vi "keccak.impl.vi"(11 "Array in":u64[](array[numeric])) -> (3 "Array out":u64[](array[numeric]))   [LabVIEW 2021]
uses:
  Step.4.5.6.7.Inputs.ctl
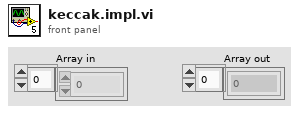
[diagram p1: front panel]
types:
  T1 = typedef "Step.4.5.6.7.Inputs.ctl" = cluster{"Left_Shift":i32, "State_Index":i32, "D_Index":i32}
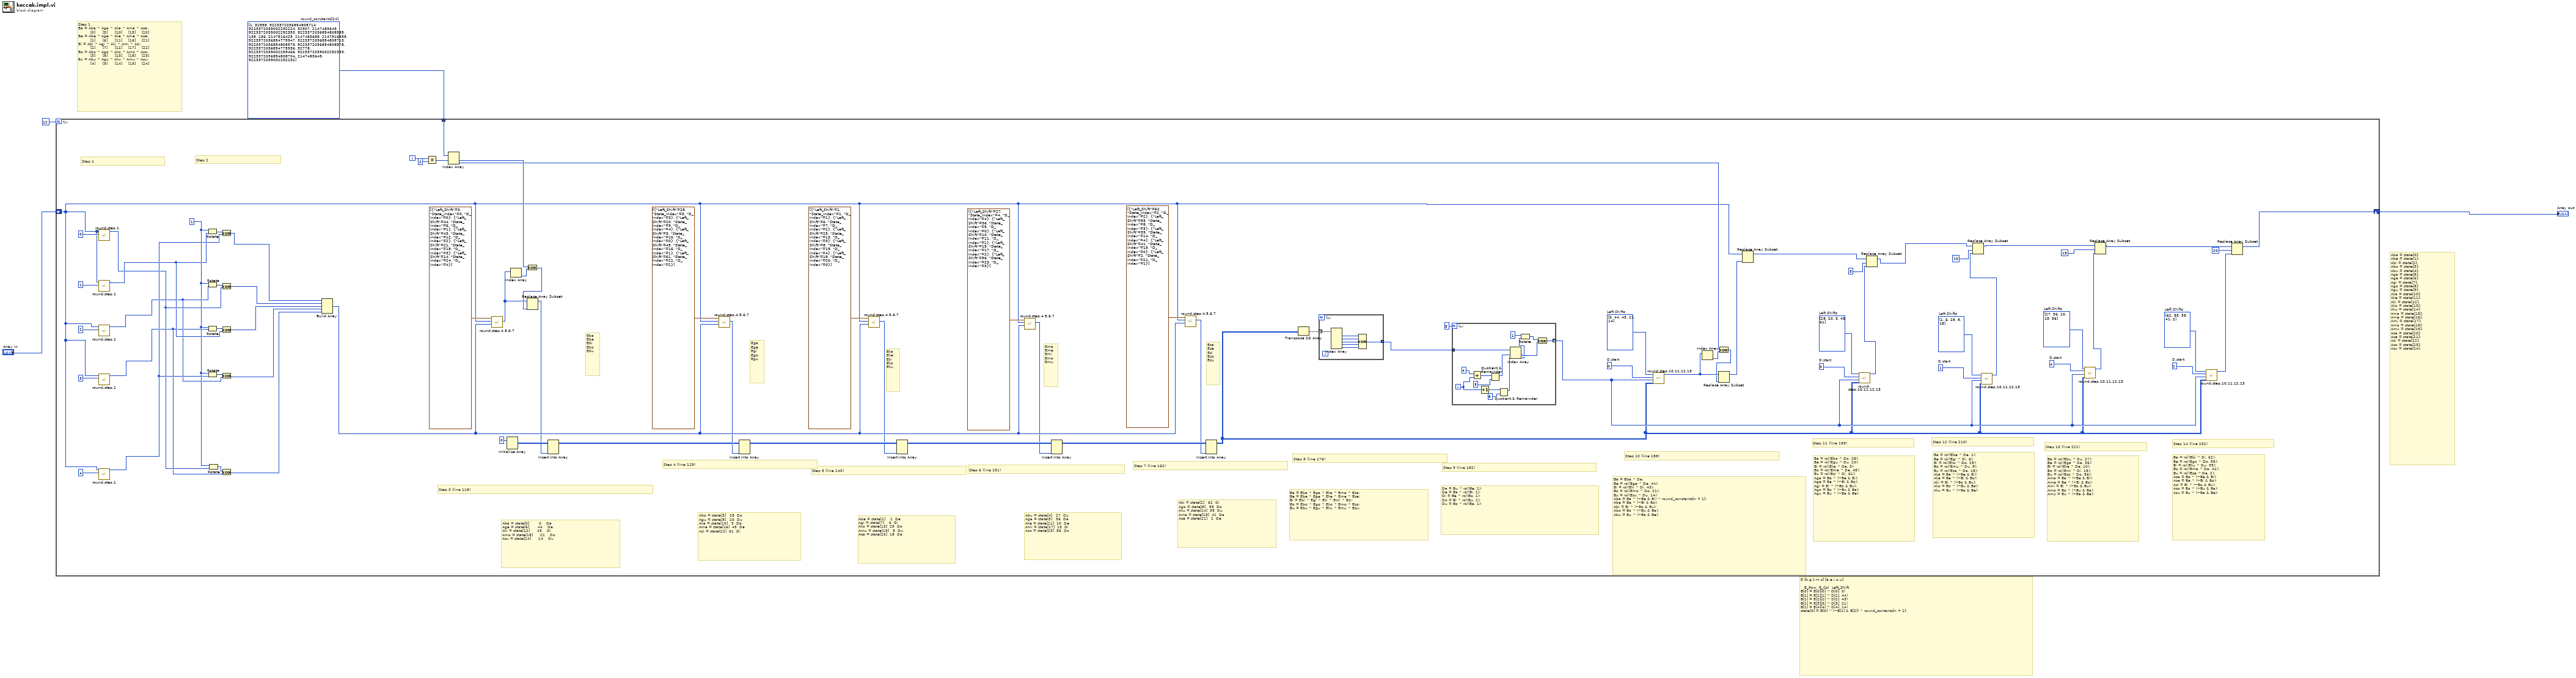
[diagram p0: block diagram]
diagram:
  w3 = u64[] [1, 32898, 9223372036854808714, 9223372039002292224, 32907, 2147483649, 9223372039002292353, 9223372036854808585, 138, 136, 2147516425, 2147483658, 2147516555, 9223372036854775947, 9223372036854808713, 9223372036854808579, 9223372036854808578, 9223372036854775936, 32778, 9223372039002259466, 9223372039002292353, 9223372036854808704, 2147483649, 9223372039002292232]  # round_constants[24]
  # "E [b,g,k,m,s] [a,e,i,o,u]\n\n   E_Row  E_Col  Left_Shift\nB[0] = E[0][0] ^ D[0], 0)\nB[1] = E[1][1] ^ D[1], 44)\nB[1] = E[2][2] ^ D[2], 43)\nB[1] = E[3][3] ^ D[3], 21)\nB[1] = E[4][4] ^ D[4], 14)\nstate[0] = B[0] ^ (~B[1] & B[2]) ^ round_contants[n + 1];"
  # "Aba = state[0];\nAbe = state[1];\nAbi = state[2];\nAbo = state[3];\nAbu = state[4];\nAga = state[5];\nAge = state[6];\nAgi = state[7];\nAgo = state[8];\nAgu = state[9];\nAka = state[10];\nAke = state[11];\nAki = state[12];\nAko = state[13];\nAku = state[14];\nAma = state[15];\nAme = state[16];\nAmi = state[17];\nAmo = state[18];\nAmu = state[19];\nAsa = state[20];\nAse = state[21];\nAsi = state[22];\nAso = state[23];\nAsu = state[24];"
  # "Step 1\nBa = Aba ^ Aga ^ Aka ^ Ama ^ Asa;\n          [0]      [5]      [10]     [15]     [20]\nBe = Abe ^ Age ^ Ake ^ Ame ^ Ase;\n          [1]      [6]      [11]     [16]     [21]\nBi = Abi ^ Agi ^ Aki ^ Ami ^ Asi;\n          [2]      [7]      [12]     [17]     [22]\nBo = Abo ^ Ago ^ Ako ^ Amo ^ Aso;\n          [3]      [8]      [13]     [18]     [23]\nBu = Abu ^ Agu ^ Aku ^ Amu ^ Asu;\n          [4]      [9]      [14]     [19]     [24]"
  n1 = for {
    N: 12 -> [_]
    tunnel: w3 -> [w65]
    shift-right: [w19] -> w4
    shift-left: "Array in" -> [w7]
    i -> [w84]
    w23 = 2  # D.start
    w22 = 4  # D.start
    w24 = i32[] [62, 55, 39, 41, 2]  # Left Shifts
    w25 = i32[] [27, 36, 10, 15, 56]  # Left Shifts
    w26 = 1  # D.start
    w27 = i32[] [1, 6, 25, 8, 18]  # Left Shifts
    w28 = 3  # D.start
    w29 = i32[] [28, 20, 3, 45, 61]  # Left Shifts
    w30 = 0  # D.start
    w35 = i32[] [0, 44, 43, 21, 14]  # Left Shifts
    w72 = i16 1 ("y")
    # "Ba = rol(Ebi ^ Di, 62);\nBe = rol(Ego ^ Do, 55);\nBi = rol(Eku ^ Du, 39);\nBo = rol(Ema ^ Da, 41);\nBu = rol(Ese ^ De, 2);\nAsa = Ba ^ (~Be & Bi);\nAse = Be ^ (~Bi & Bo);\nAsi = Bi ^ (~Bo & Bu);\nAso = Bo ^ (~Bu & Ba);\nAsu = Bu ^ (~Ba & Be);"
    # "Ba = rol(Ebu ^ Du, 27);\nBe = rol(Ega ^ Da, 36);\nBi = rol(Eke ^ De, 10);\nBo = rol(Emi ^ Di, 15);\nBu = rol(Eso ^ Do, 56);\nAma = Ba ^ (~Be & Bi);\nAme = Be ^ (~Bi & Bo);\nAmi = Bi ^ (~Bo & Bu);\nAmo = Bo ^ (~Bu & Ba);\nAmu = Bu ^ (~Ba & Be);"
    # "Step 14 (line 232)"
    # "Step 13 (line 221)"
    # "Ba = rol(Ebe ^ De, 1);\nBe = rol(Egi ^ Di, 6);\nBi = rol(Eko ^ Do, 25);\nBo = rol(Emu ^ Du, 8);\nBu = rol(Esa ^ Da, 18);\nAka = Ba ^ (~Be & Bi);\nAke = Be ^ (~Bi & Bo);\nAki = Bi ^ (~Bo & Bu);\nAko = Bo ^ (~Bu & Ba);\nAku = Bu ^ (~Ba & Be);"
    # "Step 12 (line 210)"
    # "Ba = rol(Ebo ^ Do, 28);\nBe = rol(Egu ^ Du, 20);\nBi = rol(Eka ^ Da, 3);\nBo = rol(Eme ^ De, 45);\nBu = rol(Esi ^ Di, 61);\nAga = Ba ^ (~Be & Bi);\nAge = Be ^ (~Bi & Bo);\nAgi = Bi ^ (~Bo & Bu);\nAgo = Bo ^ (~Bu & Ba);\nAgu = Bu ^ (~Ba & Be);"
    # "Step 11 (line 199)"
    # "Ba = Eba ^ Da;\nBe = rol(Ege ^ De, 44);\nBi = rol(Eki ^ Di, 43);\nBo = rol(Emo ^ Do, 21);\nBu = rol(Esu ^ Du, 14);\nAba = Ba ^ (~Be & Bi) ^ round_constants[n + 1];\nAbe = Be ^ (~Bi & Bo);\nAbi = Bi ^ (~Bo & Bu);\nAbo = Bo ^ (~Bu & Ba);\nAbu = Bu ^ (~Ba & Be);"
    # "Step 10 (line 188)"
    # "Da = Bu ^ rol(Be, 1);\nDe = Ba ^ rol(Bi, 1);\nDi = Be ^ rol(Bo, 1);\nDo = Bi ^ rol(Bu, 1);\nDu = Bo ^ rol(Ba, 1);"
    # "Step 9 (line 182)"
    # "Eba\nEbe\nEbi\nEbo\nEbu"
    # "Ega\nEge\nEgi\nEgo\nEgu"
    # "Eka\nEke\nEki\nEko\nEku"
    # "Ema\nEme\nEmi\nEmo\nEmu"
    # "Esa\nEse\nEsi\nEso\nEsu"
    # "Step 8 (line 176)"
    # "Ba = Eba ^ Ega ^ Eka ^ Ema ^ Esa;\nBe = Ebe ^ Ege ^ Eke ^ Eme ^ Ese;\nBi = Ebi ^ Egi ^ Eki ^ Emi ^ Esi;\nBo = Ebo ^ Ego ^ Eko ^ Emo ^ Eso;\nBu = Ebu ^ Egu ^ Eku ^ Emu ^ Esu;"
    # "Aba = state[0]        0    Da\nAge = state[6]       44    De\nAki = state[12]      43    Di\nAmo = state[18]      21    Do\nAsu = state[24]      14    Du"
    # "Abo = state[3]   28  Do\nAgu = state[9]   20  Du\nAka = state[10]   3  Da\nAme = state[16]  45  De\nAsi = state[22]  61  Di"
    # "Abi = state[2]   62  Di\nAgo = state[8]   55  Do\nAku = state[14]  39  Du\nAma = state[15]  41  Da\nAse = state[21]   2  De"
    # "Step 7 (line 162)"
    # "Abu = state[4]   27  Du\nAga = state[5]   36  Da\nAke = state[11]  10  De\nAmi = state[17]  15  Di\nAso = state[23]  56  Do"
    # "Step 6 (line 151)"
    # "Abe = state[1]    1  De\nAgi = state[7]    6  Di\nAko = state[13]  25  Do\nAmu = state[19]   8  Du\nAsa = state[20]  18  Da"
    # "Step 5 (line 140)"
    # "Step 4 (line 129)"
    # "Step 3 (line 118)"
    # "Step 1"
    # "Step 2"
    n2 = call "round.step.1.vi"("Numeric in"=u8 0, "Array"=w7) -> ("Numeric out"=w70:u64)  [unwired: 9 in]
    n3 = call "round.step.1.vi"("Numeric in"=u8 1, "Array"=w7) -> ("Numeric out"=w69:u64)  [unwired: 9 in]
    n4 = call "round.step.1.vi"("Numeric in"=u8 2, "Array"=w7) -> ("Numeric out"=w68:u64)  [unwired: 9 in]
    n5 = call "round.step.1.vi"("Numeric in"=u8 3, "Array"=w7) -> ("Numeric out"=w67:u64)  [unwired: 9 in]
    n6 = call "round.step.1.vi"("Numeric in"=u8 4, "Array"=w7) -> ("Numeric out"=w71:u64)  [unwired: 9 in]
    n7 = Rotate(1:w69, 2:w72) -> (0:w77:u64)
    n8 = Rotate(1:w68, 2:w72) -> (0:w76:u64)
    n9 = Rotate(1:w67, 2:w72) -> (0:w75:u64)
    n10 = Rotate(1:w71, 2:w72) -> (0:w74:u64)
    n11 = Rotate(1:w70, 2:w72) -> (0:w73:u64)
    n12 = Exclusive Or(1:w71, 2:w77) -> (0:w61:u64)
    n13 = Exclusive Or(1:w70, 2:w76) -> (0:w62:u64)
    n14 = Exclusive Or(1:w69, 2:w75) -> (0:w63:u64)
    n15 = Exclusive Or(1:w68, 2:w74) -> (0:w50:u64)
    n16 = Exclusive Or(1:w67, 2:w73) -> (0:w64:u64)
    n17 = Build Array(w61, w62, w63, w50, w64) -> (w55:u64[])
    n18 = Multiply(x=w84, y=2) -> (x*y=w66:i32)
    n19 = Index Array(array=w65, index #1=w66) -> (element #1=w52:u64, element #2=w33:u64)  [unwired: 1 in]
    n20 = call "round.step.4.5.6.7.vi"("D.in"=w55, "state[25]"=w7, "Parameters"=T1[] [{"Left_Shift"=0, "State_Index"=0, "D_Index"=0}, {"Left_Shift"=44, "State_Index"=6, "D_Index"=1}, {"Left_Shift"=43, "State_Index"=12, "D_Index"=2}, {"Left_Shift"=21, "State_Index"=18, "D_Index"=3}, {"Left_Shift"=14, "State_Index"=24, "D_Index"=4}]) -> ("E.out"=w54:u64[])  [unwired: 7 in, 1 out]
    n21 = Initialize Array(u64 0 ("element")) -> (w48:u64[][])  [unwired: 2 in]
    n22 = Index Array(array=w54) -> (element=w53:u64)  [unwired: 1 in]
    n23 = Exclusive Or(1:w53, 2:w52) -> (0:w51:u64)
    n24 = Replace Array Subset(array=w54, new element=w51) -> (w47:u64[])  [unwired: 1 in]
    n25 = Insert Into Array(array=w48, new element=w47) -> (w45:u64[][])  [unwired: 2 in]
    n26 = call "round.step.4.5.6.7.vi"("D.in"=w55, "state[25]"=w7, "Parameters"=T1[] [{"Left_Shift"=28, "State_Index"=3, "D_Index"=3}, {"Left_Shift"=20, "State_Index"=9, "D_Index"=4}, {"Left_Shift"=3, "State_Index"=10, "D_Index"=0}, {"Left_Shift"=45, "State_Index"=16, "D_Index"=1}, {"Left_Shift"=61, "State_Index"=22, "D_Index"=2}]) -> ("E.out"=w46:u64[])  [unwired: 7 in, 1 out]
    n27 = Insert Into Array(array=w45, new element=w46) -> (w44:u64[][])  [unwired: 2 in]
    n28 = call "round.step.4.5.6.7.vi"("D.in"=w55, "state[25]"=w7, "Parameters"=T1[] [{"Left_Shift"=1, "State_Index"=1, "D_Index"=1}, {"Left_Shift"=6, "State_Index"=7, "D_Index"=2}, {"Left_Shift"=25, "State_Index"=13, "D_Index"=3}, {"Left_Shift"=8, "State_Index"=19, "D_Index"=4}, {"Left_Shift"=18, "State_Index"=20, "D_Index"=0}]) -> ("E.out"=w41:u64[])  [unwired: 7 in, 1 out]
    n29 = Insert Into Array(array=w44, new element=w41) -> (w43:u64[][])  [unwired: 2 in]
    n30 = call "round.step.4.5.6.7.vi"("D.in"=w55, "state[25]"=w7, "Parameters"=T1[] [{"Left_Shift"=27, "State_Index"=4, "D_Index"=4}, {"Left_Shift"=36, "State_Index"=5, "D_Index"=0}, {"Left_Shift"=10, "State_Index"=11, "D_Index"=1}, {"Left_Shift"=15, "State_Index"=17, "D_Index"=2}, {"Left_Shift"=56, "State_Index"=23, "D_Index"=3}]) -> ("E.out"=w40:u64[])  [unwired: 7 in, 1 out]
    n31 = Insert Into Array(array=w43, new element=w40) -> (w42:u64[][])  [unwired: 2 in]
    n32 = call "round.step.4.5.6.7.vi"("D.in"=w55, "state[25]"=w7, "Parameters"=T1[] [{"Left_Shift"=62, "State_Index"=2, "D_Index"=2}, {"Left_Shift"=55, "State_Index"=8, "D_Index"=3}, {"Left_Shift"=39, "State_Index"=14, "D_Index"=4}, {"Left_Shift"=41, "State_Index"=15, "D_Index"=0}, {"Left_Shift"=2, "State_Index"=21, "D_Index"=1}]) -> ("E.out"=w39:u64[])  [unwired: 7 in, 1 out]
    n33 = Insert Into Array(array=w42, new element=w39) -> (w20:u64[][])  [unwired: 2 in]
    n34 = Transpose 2D Array(2D array=w20) -> (transposed array=w38:u64[][])
    n35 = for {
      tunnel: w38 -> [w105] mode=indexing
      tunnel: [w99] -> w36 mode=indexing
      n36 = Index Array(array=w105) -> (element #1=w104:u64, element #2=w103:u64, element #3=w102:u64, element #4=w101:u64, element #5=w100:u64)  [unwired: 5 in]
      n37 = Compound Arithmetic op=XOR(w104, w103, w102, w101, w100) -> (w99:u64)
    }
    n38 = for {
      N: 5 -> [_]
      tunnel: w36 -> [w96]
      tunnel: [w95] -> w21 mode=indexing
      i -> [w93]
      n39 = Add(x=4, y=w93) -> (x+y=w89:i32)
      n40 = Increment(x=w93) -> (x+1=w86:i32)
      n41 = Quotient & Remainder(x=w89, y=5 ("x")) -> (x-y*floor(x/y)=w87:i32)  [unwired: 1 out]
      n42 = Quotient & Remainder(x=w86, y=5 ("x")) -> (x-y*floor(x/y)=w90:i32)  [unwired: 1 out]
      n43 = Index Array(array=w96, index #1=w87, index #2=w90) -> (element #1=w92:u64, element #2=w91:u64)
      n44 = Rotate(1:w91, 2:i16 1 ("y")) -> (0:w98:u64)
      n45 = Exclusive Or(1:w92, 2:w98) -> (0:w95:u64)
    }
    n46 = call "round.step.10.11.12.13.vi"("E.Values"=w20, "D.Values"=w21, "D.Offsets"=w30, "Left Shifts"=w35) -> ("Final.A.Out"=w32:u64[])  [unwired: 7 in]
    n47 = Index Array(array=w32) -> (element=w34:u64)  [unwired: 1 in]
    n48 = Exclusive Or(1:w34, 2:w33) -> (0:w31:u64)
    n49 = Replace Array Subset(array=w32, new element=w31) -> (w5:u64[])  [unwired: 1 in]
    n50 = Replace Array Subset(array=w7, new element=w5) -> (w6:u64[])  [unwired: 1 in]
    n51 = call "round.step.10.11.12.13.vi"("E.Values"=w20, "D.Values"=w21, "D.Offsets"=w28, "Left Shifts"=w29) -> ("Final.A.Out"=w9:u64[])  [unwired: 7 in]
    n52 = Replace Array Subset(array=w6, new element=w9, index=5) -> (w8:u64[])
    n53 = call "round.step.10.11.12.13.vi"("E.Values"=w20, "D.Values"=w21, "D.Offsets"=w26, "Left Shifts"=w27) -> ("Final.A.Out"=w12:u64[])  [unwired: 7 in]
    n54 = Replace Array Subset(array=w8, new element=w12, index=10) -> (w11:u64[])
    n55 = call "round.step.10.11.12.13.vi"("E.Values"=w20, "D.Values"=w21, "D.Offsets"=w22, "Left Shifts"=w25) -> ("Final.A.Out"=w15:u64[])  [unwired: 7 in]
    n56 = Replace Array Subset(array=w11, new element=w15, index=15) -> (w14:u64[])
    n57 = call "round.step.10.11.12.13.vi"("E.Values"=w20, "D.Values"=w21, "D.Offsets"=w23, "Left Shifts"=w24) -> ("Final.A.Out"=w17:u64[])  [unwired: 7 in]
    n58 = Replace Array Subset(array=w14, new element=w17, index=20) -> (w19:u64[])
  }
  "Array out" <- w4
